vi "CRYHarmonic cursors4.vi"(0 "Cursor List in":T1(array[cluster]) {"Cursor Position"."Cursor Y" format="%.2f"; "Cursor Position"."Cursor X" format="%.2f"}, 1 "Log data":bool, 3 "dB ref":dbl format="%.2f", 5 "Harm. cursor on":bool, 7 "window constants":cluster{"eq noise BW":dbl, "coherent gain":dbl}={"eq noise BW"=1.0, "coherent gain"=1.0} {"coherent gain" format="%.2f"; "eq noise BW" format="%.2f"}, 8 "Estimated power":dbl format="%.2f", 9 "df":dbl format="%.2f", 11 "n f points":i32, 12 "Cursor free":bool, 13 "Power spectrum":dbl[](array[numeric]) format="%.2f", 14 "Spectrum y":dbl[](array[numeric]) format="%.2f", 15 "Estimated freq.":dbl format="%.2f") -> (4 "Cursor List out":T1(array[cluster]) {"Cursor Position"."Cursor Y" format="%.2f"; "Cursor Position"."Cursor X" format="%.2f"}, 6 "THD (%)":dbl format="%.2f", 10 "Cursor locked mode":u32)   [LabVIEW 2013]
uses:
  <vilib>/Analysis/NI_AALPro.lvlib
panel:
  in  "help":bool=TRUE
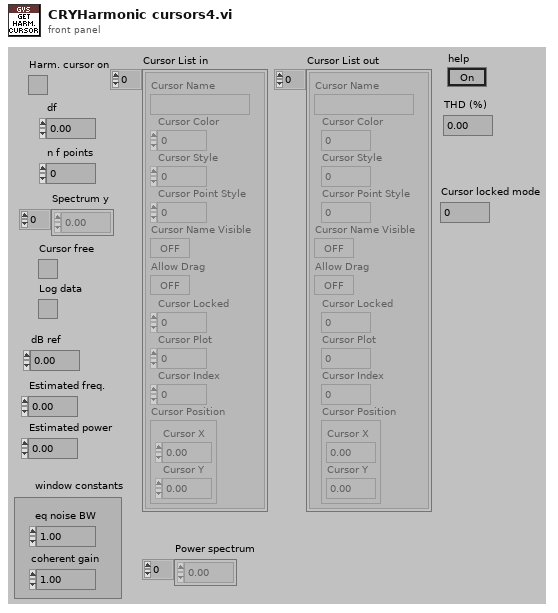
[diagram p1: front panel]
types:
  T1 = cluster{"Cursor Name":string, "Cursor Color":u32, "Cursor Style":u8, "Cursor Point Style":u8, "Cursor Name Visible":bool, "Allow Drag":bool, "Cursor Locked":u32, "Cursor Plot":u32, "Cursor Index":i32, "Cursor Position":cluster{"Cursor X":dbl, "Cursor Y":dbl}}[]
  T2 = cluster{"Cursor Name":string, "Cursor Color":u32, "Cursor Style":u8, "Cursor Point Style":u8, "Cursor Name Visible":bool, "Allow Drag":bool, "Cursor Locked":u32, "Cursor Plot":u32, "Cursor Index":i32, "Cursor Position":cluster{"Cursor X":dbl, "Cursor Y":dbl}}
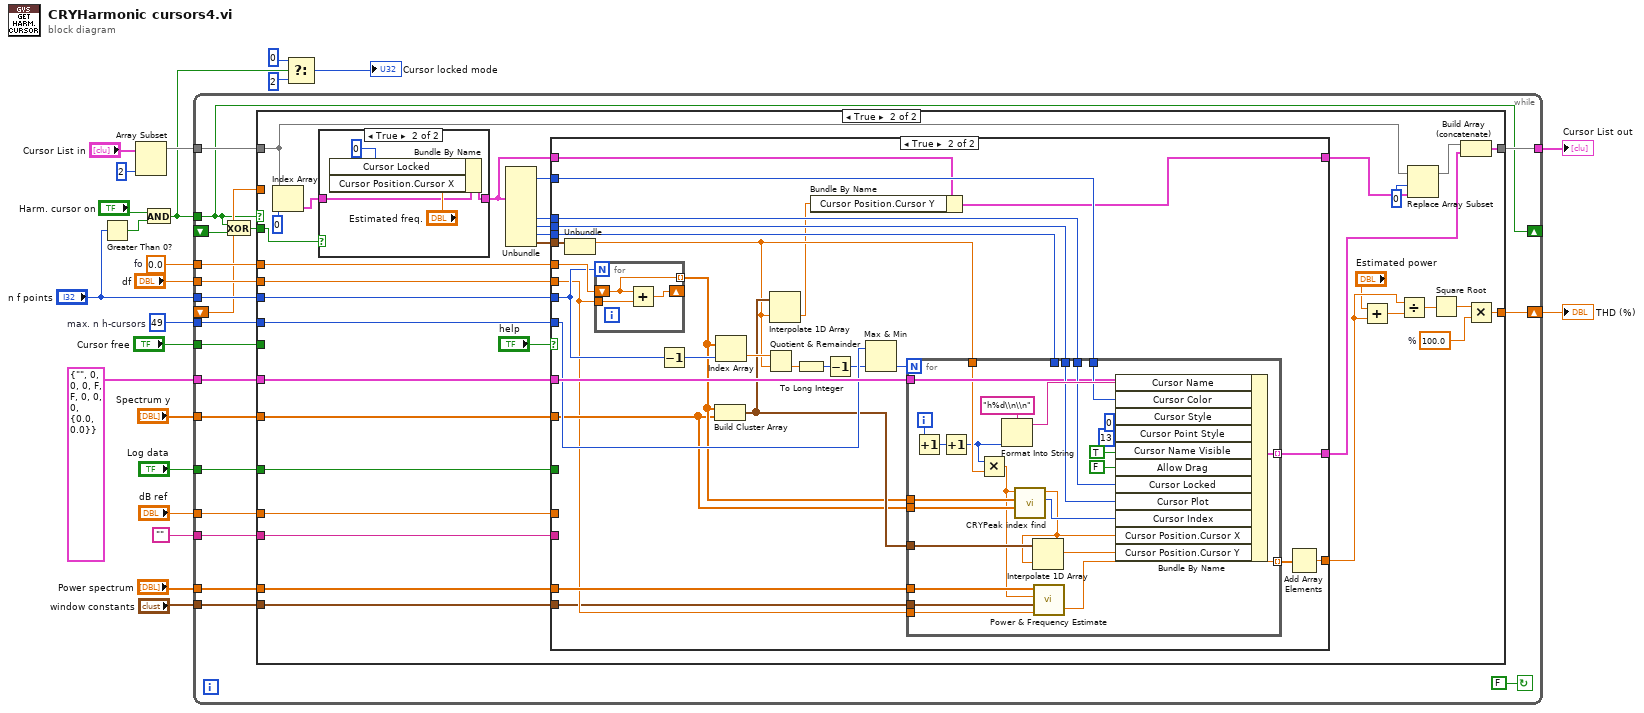
[diagram p0: block diagram]
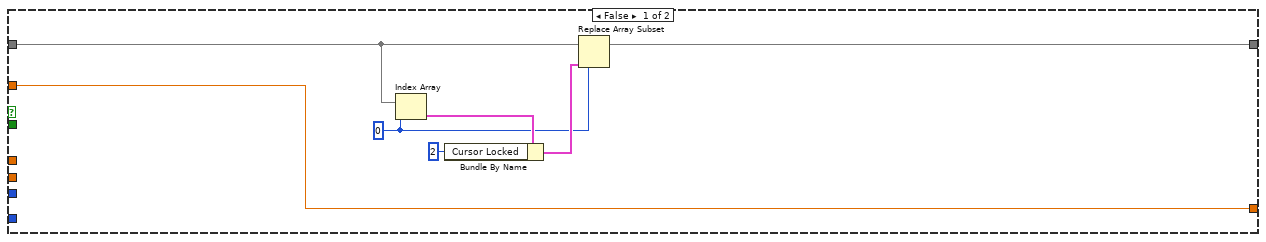
[diagram p2: hidden frame]
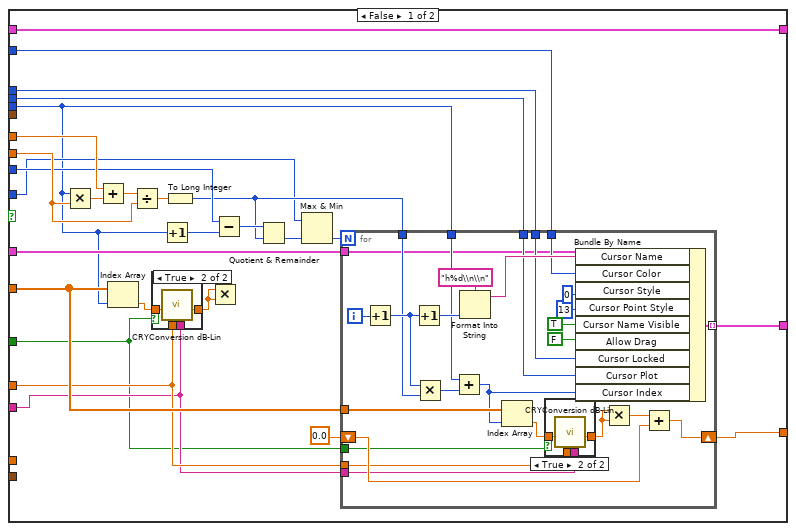
[diagram p4: hidden frame]
diagram:
  w13 = 49  # max. n h-cursors
  w19 = 0.0  # fo
  n1 = Greater Than 0?(x="n f points") -> (x > 0?=w15:bool)
  n2 = Array Subset(array="Cursor List in", length=2 ("Array Length")) -> (w20:T1)  [unwired: 1 in]
  n3 = And(x="Harm. cursor on", y=w15) -> (x .and. y?=w6:bool)
  n4 = while {
    tunnel: "window constants" -> [w25]
    tunnel: "Power spectrum" -> [w26]
    shift-left: _ -> [w28]
    shift-right: [w29] -> _
    tunnel: "" -> [w30]
    tunnel: "dB ref" -> [w31]
    tunnel: "Log data" -> [w32]
    shift-left: _ -> [w33]
    shift-right: [w34] -> w10
    tunnel: "Spectrum y" -> [w35]
    tunnel: "Cursor free" -> [w36]
    tunnel: w13 -> [w37]
    tunnel: w6 -> [w29]
    tunnel: "n f points" -> [w38]
    tunnel: T2 {"Cursor Name"="", "Cursor Color"=0, "Cursor Style"=0, "Cursor Point Style"=0, "Cursor Name Visible"=FALSE, "Allow Drag"=FALSE, "Cursor Locked"=0, "Cursor Plot"=0, "Cursor Index"=0, "Cursor Position"={"Cursor X"=0.0, "Cursor Y"=0.0}} ("Write Attribute") -> [w39]
    tunnel: "df" -> [w40]
    tunnel: w19 -> [w41]
    tunnel: w20 -> [w42]
    tunnel: [w43] -> w23
    stop <- FALSE continue-if-true
    n5 = Exclusive Or(1:w28, 2:w29) -> (0:w27:bool)
    n6 = case shown="True" w29 {
      tunnel: [w44 w75] -> w43
      tunnel: w42 -> [w45 w56]
      tunnel: w41 -> [_ w83]
      tunnel: w40 -> [_ w82]
      tunnel: w38 -> [_ w81]
      tunnel: w39 -> [_ w76]
      tunnel: w37 -> [_ w74]
      tunnel: w36 -> [_ _]
      tunnel: w35 -> [_ w73]
      tunnel: [w50 w66] -> w34
      tunnel: w33 -> [w50 _]
      tunnel: w32 -> [_ w65]
      tunnel: w31 -> [_ w64]
      tunnel: w30 -> [_ w63]
      tunnel: w27 -> [_ w61]
      tunnel: w26 -> [_ w53]
      tunnel: w25 -> [_ w52]
      frame False {
        w46 = 0 ("Index")
        n7 = Index Array(array=w45, index=w46) -> (element=w48:T2)
        n8 = Bundle By Name(cluster=w48, "Cursor Locked"=u32 2 ("Bundle Element")) -> (w47:T2)
        n9 = Replace Array Subset(array=w45, new element=w47, index=w46) -> (w44:T1)
      }
      frame True {
        w68 = 100.0  # %
        n10 = Index Array(array=w56, index=0 ("Index")) -> (element=w62:T2)
        n11 = case shown="True" w61 {
          tunnel: w62 -> [w85 w88]
          tunnel: [w85 w86] -> w59
          frame False {
          }
          frame True {
            n12 = Bundle By Name(cluster=w88, "Cursor Locked"=u32 0 ("Bundle Element"), "Cursor Position.Cursor X"="Estimated freq.") -> (w86:T2)
          }
        }
        n13 = Unbundle(w59) -> ("Cursor Color"=w80:u32, "Cursor Locked"=w79:u32, "Cursor Plot"=w78:u32, "Cursor Index"=w77:i32, "Cursor Position"=w72:cluster{"Cursor X":dbl, "Cursor Y":dbl})  [unwired: 5 out]
        n14 = case shown="True" "help" {
          tunnel: w83 -> [w116 w171]
          tunnel: w82 -> [w113 w155]
          tunnel: w81 -> [w111 w170]
          tunnel: w80 -> [w108 w181]
          tunnel: w79 -> [w107 w180]
          tunnel: w78 -> [w106 w179]
          tunnel: w77 -> [w96 w173]
          tunnel: w76 -> [w104 w178]
          tunnel: [w101 w175] -> w54
          tunnel: w74 -> [w100 w174]
          tunnel: w73 -> [w97 w157]
          tunnel: w72 -> [_ w172]
          tunnel: [w98 w164] -> w70
          tunnel: w65 -> [w91 _]
          tunnel: w64 -> [w93 _]
          tunnel: w63 -> [w92 _]
          tunnel: w59 -> [w90 w160]
          tunnel: [w90 w159] -> w57
          tunnel: w53 -> [_ w156]
          tunnel: w52 -> [_ w154]
          frame False {
            n15 = Multiply(x=w96, y=w113) -> (x*y=w115:dbl)
            n16 = Add(x=w116, y=w115) -> (x+y=w114:dbl)
            n17 = Index Array(array=w97, index=w96) -> (element=w95:dbl)
            n18 = Divide(x=w114, y=w113) -> (x/y=w112:dbl)
            n19 = case shown="True" w91 {
              tunnel: w95 -> [w117 w121]
              tunnel: [w117 w120] -> w94
              tunnel: w93 -> [_ w119]
              tunnel: w92 -> [_ w118]
              frame False {
              }
              frame True {
                n20 = call "CRYConversion dB-Lin.vi"("unit prefix"=w118, "dB ref."=w119, "Log In"=w121) -> ("Lin Out"=w120:dbl)  [unwired: 3 in, 3 out]
              }
            }
            n21 = Increment(x=w96) -> (x+1=w110:i32)
            n22 = To Long Integer(number=w112) -> (32bit integer=w105:i32)
            n23 = Multiply(x=w94, y=w94) -> ()  [unwired: 1 out]
            n24 = Subtract(x=w111, y=w110) -> (x-y=w109:i32)
            n25 = Quotient & Remainder(x=w109, y=w105) -> (floor(x/y)=w103:i32)  [unwired: 1 out]
            n26 = Max & Min(x=w100, y=w103) -> (min(x,y)=w102:i32)  [unwired: 1 out]
            n27 = for {
              N: w102 -> [_]
              tunnel: w108 -> [w146]
              tunnel: w107 -> [w141]
              tunnel: w106 -> [w140]
              tunnel: w105 -> [w136]
              tunnel: w96 -> [w135]
              tunnel: w104 -> [w133]
              tunnel: [w132] -> w101 mode=indexing
              shift-right: [w127] -> w98
              shift-left: 0.0 -> [w128]
              tunnel: w97 -> [w131]
              tunnel: w93 -> [w124]
              tunnel: w92 -> [w123]
              tunnel: w91 -> [w122]
              i -> [w139]
              n28 = Increment(x=w139) -> (x+1=w137:i32)
              n29 = Increment(x=w137) -> (x+1=w138:i32)
              n30 = Multiply(x=w137, y=w136) -> (x*y=w134:i32)
              n31 = Add(x=w135, y=w134) -> (x+y=w130:i32)
              n32 = Format Into String(format string="h%d\\n\\n", w138) -> (resulting string=w147:string)  [unwired: 2 in, 1 out]
              n33 = Index Array(array=w131, index=w130) -> (element=w126:dbl)
              n34 = case shown="True" w122 {
                tunnel: w126 -> [w149 w153]
                tunnel: [w149 w152] -> w125
                tunnel: w124 -> [_ w151]
                tunnel: w123 -> [_ w150]
                frame False {
                }
                frame True {
                  n35 = call "CRYConversion dB-Lin.vi"("unit prefix"=w150, "dB ref."=w151, "Log In"=w153) -> ("Lin Out"=w152:dbl)  [unwired: 3 in, 3 out]
                }
              }
              n36 = Bundle By Name(cluster=w133, "Cursor Name"=w147, "Cursor Color"=w146, "Cursor Style"=u8 0 ("Bundle Element"), "Cursor Point Style"=u8 13 ("Bundle Element"), "Cursor Name Visible"=TRUE ("Bundle Element"), "Allow Drag"=FALSE ("Bundle Element"), "Cursor Locked"=w141, "Cursor Plot"=w140, "Cursor Index"=w130) -> (w132:T2)
              n37 = Multiply(x=w125, y=w125) -> (x*y=w129:dbl)
              n38 = Add(x=w129, y=w128) -> (x+y=w127:dbl)
            }
          }
          frame True {
            n39 = Unbundle(w172) -> ("Cursor X"=w162:dbl)  [unwired: 1 out]
            n40 = for {
              N: w170 -> [_]
              shift-right: [w183] -> _
              shift-left: w171 -> [w182]
              tunnel: w155 -> [w184]
              tunnel: [w182] -> w158 mode=indexing
              n41 = Add(x=w182, y=w184) -> (x+y=w183:dbl)
            }
            n42 = Decrement(x=w170) -> (x-1=w169:i32)
            n43 = Build Cluster Array(w158, w157) -> (w163:cluster{"fo":dbl, "Numeric":dbl}[])
            n44 = Index Array(array=w158, index=w169) -> (element=w168:dbl)
            n45 = Quotient & Remainder(x=w168, y=w162) -> (floor(x/y)=w177:dbl)  [unwired: 1 out]
            n46 = Interpolate 1D Array(1:w162, 2:w163) -> (0:w161:dbl)
            n47 = To Long Integer(number=w177) -> (32bit integer=w167:i32)
            n48 = Bundle By Name(cluster=w160, "Cursor Position.Cursor Y"=w161) -> (w159:T2)
            n49 = Decrement(x=w167) -> (x-1=w166:i32)
            n50 = Max & Min(x=w174, y=w166) -> (min(x,y)=w176:i32)  [unwired: 1 out]
            n51 = for {
              N: w176 -> [_]
              tunnel: w181 -> [w208]
              tunnel: w180 -> [w203]
              tunnel: w179 -> [w202]
              tunnel: w162 -> [w198]
              tunnel: w178 -> [w200]
              tunnel: [w199] -> w175 mode=indexing
              tunnel: w173 -> [_]
              tunnel: w163 -> [w195]
              tunnel: [w187] -> w165 mode=indexing
              tunnel: w158 -> [w193]
              tunnel: w157 -> [w192]
              tunnel: w156 -> [w190]
              tunnel: w155 -> [w189]
              tunnel: w154 -> [w188]
              i -> [w201]
              n52 = Increment(x=w201) -> (x+1=w197:i32)
              n53 = Increment(x=w197) -> (x+1=w196:i32)
              n54 = Multiply(x=w196, y=w198) -> (x*y=w185:dbl)
              n55 = Format Into String(format string="h%d\\n\\n", w196) -> (resulting string=w209:string)  [unwired: 2 in, 1 out]
              n56 = call "CRYPeak index find.vi"("Y array"=w192, "X array"=w193, "X value"=w185) -> ("Peak index of array"=w194:i32, "X of peak point"=w186:dbl)  [unwired: 7 out]
              n57 = Interpolate 1D Array(1:w186, 2:w195) -> (0:w191:dbl)
              n58 = call <vilib>:"Power & Frequency Estimate.vi"("df"=w189, "window constants"=w188, "peak frequency (max)"=w185, "Power Spectrum (V^2 rms)"=w190) -> ("est power peak"=w187:dbl)  [unwired: 1 in, 2 out]
              n59 = Bundle By Name(cluster=w200, "Cursor Name"=w209, "Cursor Color"=w208, "Cursor Style"=u8 0 ("Bundle Element"), "Cursor Point Style"=u8 13 ("Bundle Element"), "Cursor Name Visible"=TRUE ("Bundle Element"), "Allow Drag"=FALSE ("Bundle Element"), "Cursor Locked"=w203, "Cursor Plot"=w202, "Cursor Index"=w194, "Cursor Position.Cursor X"=w186, "Cursor Position.Cursor Y"=w191) -> (w199:T2)
            }
            n60 = Add Array Elements(numeric array=w165) -> (sum=w164:dbl)
          }
        }
        n61 = Add(x="Estimated power", y=w70) -> (x+y=w71:dbl)
        n62 = Divide(x=w70, y=w71) -> (x/y=w69:dbl)
        n63 = Replace Array Subset(array=w56, new element=w57, index=0 ("Index")) -> (w55:T1)
        n64 = Square Root(x=w69) -> (sqrt(x)=w67:dbl)
        n65 = Build Array (concatenate)(w55, w54) -> (w75:T1)
        n66 = Multiply(x=w67, y=w68) -> (x*y=w66:dbl)
      }
    }
  }
  "Cursor List out" <- w23
  "THD (%)" <- w10
  n67 = Select(t=u32 0 ("Cursor locked mode"), s=w6, f=u32 2 ("Cursor locked mode")) -> (s? t:f=→"Cursor locked mode":u32)
